vi "Convert.vi"(1 "Numeric In":dbl) -> (0 "Numeric Out":dbl)   [LabVIEW 2015]
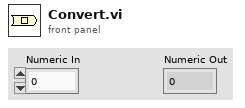
[diagram p1: front panel]
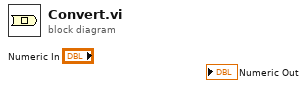
[diagram p0: block diagram]
diagram:
